vi "Normalize.vi"(0 "Normalization":bool=TRUE, 2 "Pulse signal in":dbl[](array[numeric])) -> (6 "Pulse signal out":dbl[](array[numeric]))   [LabVIEW 2018]
panel:
  out "Pulse signal in graph out":dbl[](graph)
  out "Pulse signal in graph":dbl[](graph)
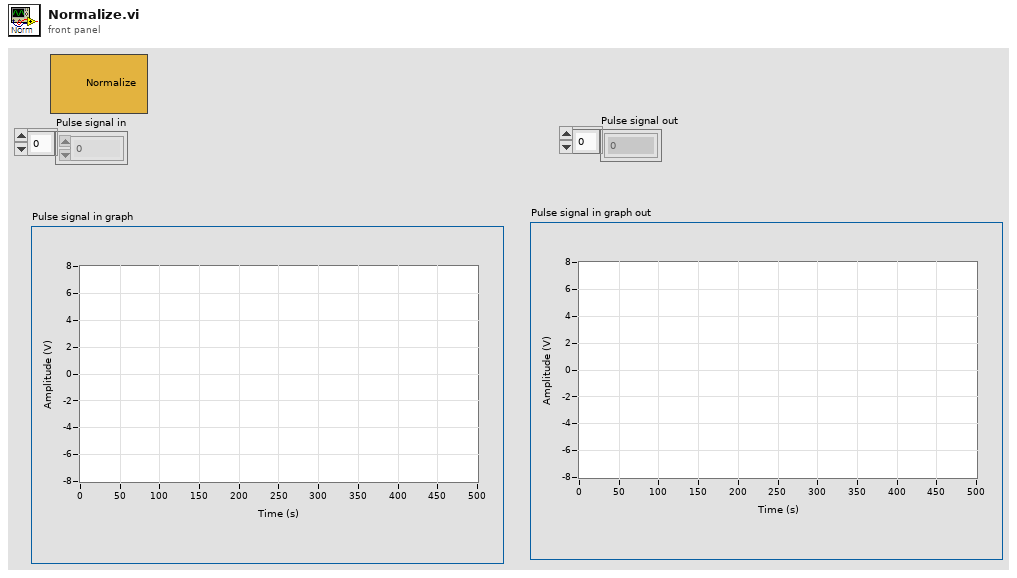
[diagram p1: front panel]
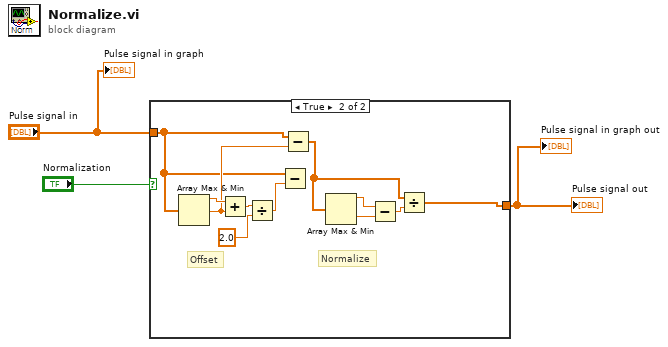
[diagram p0: block diagram]
diagram:
  n1 = case shown="True" "Normalization" {
    tunnel: "Pulse signal in" -> [w4 w7]
    tunnel: [w4 w6] -> w2
    frame False {
    }
    frame True {
      # "Normalize"
      # "Offset"
      n2 = Array Max & Min(array=w7) -> (max value=w12:dbl, min value=w8:dbl)  [unwired: 2 out]
      n3 = Add(x=w12, y=w8) -> (x+y=w11:dbl)
      n4 = Divide(x=w11, y=2.0) -> (x/y=w9:dbl)
      n5 = Subtract(x=w7, y=w9) -> ()  [unwired: 1 out]
      n6 = Subtract(x=w7, y=w8) -> (x-y=w5:dbl[])
      n7 = Array Max & Min(array=w5) -> (max value=w15:dbl, min value=w14:dbl)  [unwired: 2 out]
      n8 = Subtract(x=w15, y=w14) -> (x-y=w13:dbl)
      n9 = Divide(x=w5, y=w13) -> (x/y=w6:dbl[])
    }
  }
  "Pulse signal out" <- w2
  "Pulse signal in graph out" <- w2
  "Pulse signal in graph" <- "Pulse signal in"
